vi "Spreadsheet Storage.vi"() -> ()   [LabVIEW 2015]
uses:
  <vilib>/Utility/file.llb/Write Delimited Spreadsheet (DBL).vi
panel:
  in  "Waveform Parameters":T1
  in  "Digitizing Parameters":T2
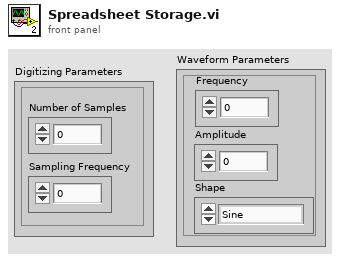
[diagram p1: front panel]
types:
  T1 = cluster{"Frequency":dbl, "Amplitude":dbl, "Shape":enum16{"Sine", "Cosine", "DC Level", "Square", "User-Defined"}}
  T2 = cluster{"Number of Samples":i32, "Sampling Frequency":dbl}
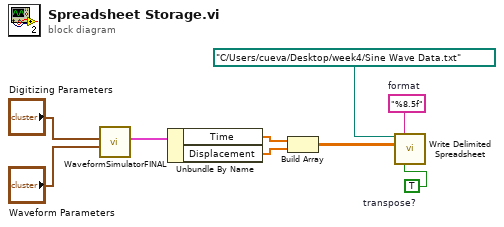
[diagram p0: block diagram]
diagram:
  w5 = "%8.5f"  # format
  w9 = TRUE  # transpose?
  n1 = call "WaveformSimulatorFINAL.vi"("Waveform Parameters"="Waveform Parameters", "Digitizing Parameters"="Digitizing Parameters") -> ("Waveform Output"=w2:cluster{"Time":dbl[], "Displacement":dbl[]})  [unwired: 9 in]
  n2 = Unbundle By Name(w2) -> ("Time"=w8:dbl[], "Displacement"=w7:dbl[])
  n3 = Build Array "Build Array"(w8, w7) -> (w6:dbl[][])
  n4 = call-poly <vilib>:"Write Delimited Spreadsheet.vi"("file path (dialog if empty)"=path "C:/Users/cueva/Desktop/week4/Sine Wave Data.txt", "format (%.3f)"=w5, "2D data"=w6, "transpose? (F)"=w9) -> ()  [unwired: 10 in, 2 out]
